vi "TimeInterpVariant_CleanUp.vi"(11 "in TimeInterpVariant":T1) -> (0 "Error":bool, 3 "out TimeInterpVariant":T1)   [LabVIEW 2019, in "Trajectory_Library.lvlib"]
doc: "Removes samples older than our current history size.\n\nInputs:\n - In TimeInterpPose2d -- Input data cluster.\n\nOutputs:\n - Out TimeInterpPose2d -- Updated data cluster.\n - Error -- Returns TRUE if an error occured."
uses:
  Trajectory_Library.lvlib
  <vilib>/gmath/NI_Gmath.lvlib
  TypeDef/TIME_INTERPOLATABLE_VARIANT.ctl
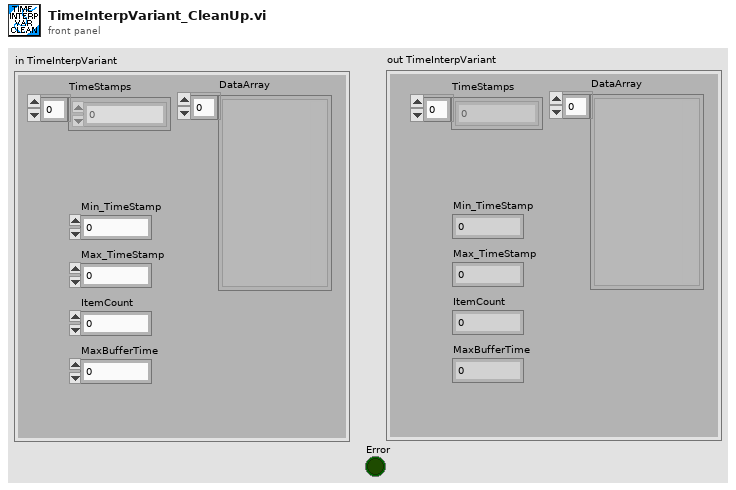
[diagram p1: front panel]
types:
  T1 = typedef "Trajectory_Library.lvlib/TIME_INTERPOLATABLE_VARIANT.ctl" = cluster{"TimeStamps":dbl[], "DataArray":variant[], "Min_TimeStamp":dbl, "Max_TimeStamp":dbl, "ItemCount":i32, "MaxBufferTime":dbl}
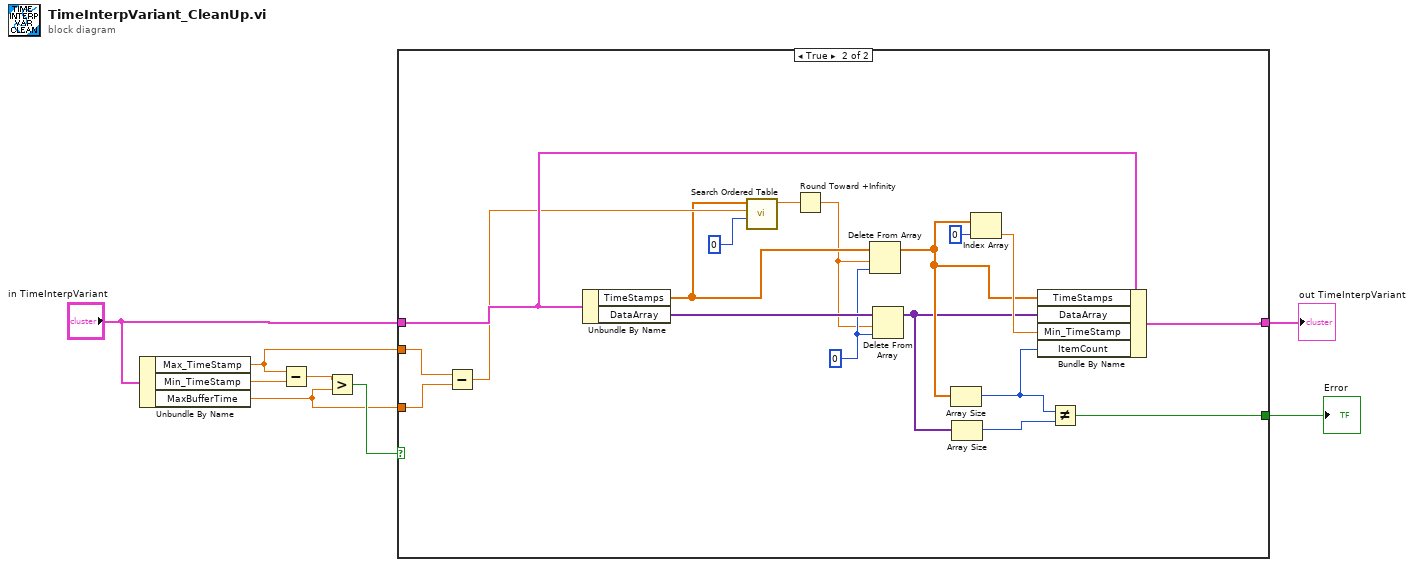
[diagram p0: block diagram]
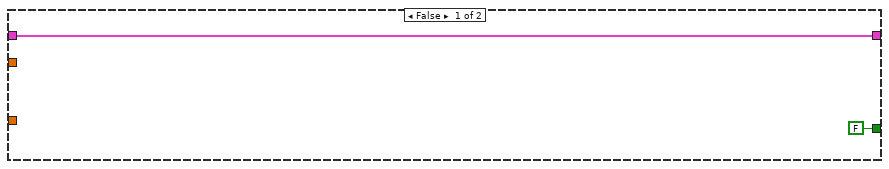
[diagram p2: hidden frame]
diagram:
  n1 = Unbundle By Name("in TimeInterpVariant") -> ("Max_TimeStamp"=w3:dbl, "Min_TimeStamp"=w6:dbl, "MaxBufferTime"=w2:dbl)
  n2 = Subtract(x=w3, y=w6) -> (x-y=w5:dbl)
  n3 = Greater?(x=w5, y=w2) -> (0:w4:bool)
  n4 = case shown="True" w4 {
    tunnel: "in TimeInterpVariant" -> [w10 w26]
    tunnel: [w10 w24] -> w8
    tunnel: w3 -> [_ w28]
    tunnel: w2 -> [_ w27]
    tunnel: [FALSE w23] -> w1
    frame False {
    }
    frame True {
      w18 = 0 ("index")
      n5 = Subtract(x=w28, y=w27) -> (x-y=w25:dbl)
      n6 = Unbundle By Name(w26) -> ("TimeStamps"=w21:dbl[], "DataArray"=w20:variant[])
      n7 = call <vilib>:"Search Ordered Table.vi"("starting index"=0, "x value"=w25, "ordered x array"=w21) -> ("fractional index"=w19:dbl)  [unwired: 8 in]
      n8 = Round Toward +Infinity(x=w19) -> (ceil(x): smallest int >= x=w17:dbl)
      n9 = Delete From Array(array=w21, length=w17, index=w18) -> (array with subset deleted=w14:dbl[])  [unwired: 1 out]
      n10 = Delete From Array(array=w20, length=w17, index=w18) -> (array with subset deleted=w13:variant[])  [unwired: 1 out]
      n11 = Array Size(array=w14) -> (size(s)=w12:i32)
      n12 = Array Size(array=w13) -> (size(s)=w11:i32)
      n13 = Index Array(array=w14, index=0) -> (element=w15:dbl)
      n14 = Bundle By Name(cluster=w26, "TimeStamps"=w14, "DataArray"=w13, "Min_TimeStamp"=w15, "ItemCount"=w12) -> (w24:T1)
      n15 = Not Equal?(x=w12, y=w11) -> (x != y?=w23:bool)
    }
  }
  "out TimeInterpVariant" <- w8
  "Error" <- w1
